vi "Teleop.vi"(10 "Match Info":T1={"Autonomous Elapsed Seconds"=0.0, "TeleOp Elapsed Seconds"=0.0, "Disabled Elapsed Seconds"=0.0, "Visited Autonomous"=FALSE, "Visited TeleOp"=FALSE, "Visited Disabled"=FALSE, "Autonomous Settings"={"Autonomous Style"=enum."Independent", "VI Refnum"=refnum}}, 11 "Call Context":T2) -> ()   [LabVIEW 2017]
doc: "This VI is called for each TeleOp packet received from the DS where the robot is not disabled. It is often used to read from the joysticks and update I/O or to update setpoints for timed control loops. It should complete and return within 20 milliseconds or it may miss DS packets."
uses:
  <vilib>/Rock Robotics/WPI/DriverStation/WPI_DriverStationDerivedRobotMode.ctl
  <vilib>/Rock Robotics/WPI/DriverStation/WPI_DriverStationMatch Info.ctl
  Climb Controls.ctl
  Cube Manipulation Manual Controls.ctl
  Cube Manipulation Controls.ctl
  <vilib>/Rock Robotics/WPI/ThirdParty/Phoenix-LabVIEW/Motor Controller/Controls/CTRE_Phoenix_MotorControl_ControlMode.ctl
  Robot Global Data.vi
  <vilib>/Rock Robotics/WPI/Utilities/WPI_GetSetVariantRefNum.vi
  <vilib>/Rock Robotics/WPI/Solenoid/Deprecated/WPI_SolenoidSetBool.vi
  <vilib>/Rock Robotics/WPI/Solenoid/Deprecated/WPI_SolenoidGetBool.vi
panel:
  out "Ramp Tail":bool
  out "Ramp Drop":bool
  in  "Carrage Contiunous voltage":dbl=-1.0
  in  "Swerve Debug Mode":bool
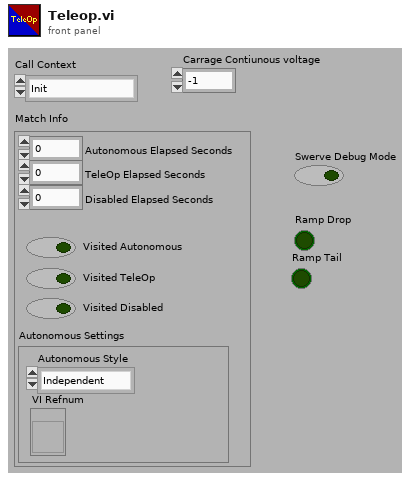
[diagram p1: front panel]
types:
  T1 = typedef "WPI_DriverStationMatch Info.ctl" = cluster{"Autonomous Elapsed Seconds":dbl, "TeleOp Elapsed Seconds":dbl, "Disabled Elapsed Seconds":dbl, "Visited Autonomous":bool, "Visited TeleOp":bool, "Visited Disabled":bool, "Autonomous Settings":cluster{"Autonomous Style":enum16{"Iterative", "Independent"}, "VI Refnum":refnum<vi>}}
  T2 = typedef "WPI_DriverStationDerivedRobotMode.ctl" = enum16{"Init", "Execute", "Stop"}
  T3 = typedef "Cube Manipulation Controls.ctl" = cluster{"Intake Sequence":bool, "Switch Position":bool, "Scale Position Low":bool, "Scale Position Mid":bool, "Scale Position High":bool, "Re-adjust Grip":bool, "Manual Mode":bool, "Manual Toggle Long":bool, "Manual Toggle Short":bool, "Eject Cube":bool, "Manual Lift Control":bool, "Exchange Sequence":bool, "Open Intk Short 4 Intk":bool, "Slow Eject":bool}
  T4 = typedef "Cube Manipulation Manual Controls.ctl" = cluster{"Extend Long Solinoid":bool, "Retract Long Solinoid":bool, "Extend Short Solinoid":bool, "Retract Short Solinoid":bool, "Override Lift Control":bool, "Override Intake Control":bool, "Clear Intake Area":bool}
  T5 = typedef "Climb Controls.ctl" = cluster{"Drop Ramps":bool, "Lift to Climb":bool, "Attach Hooks":bool, "Extend Ramp Tail":bool, "Climb Output":dbl, "Lift to Cube Hold":bool, "Retract Ramp Tail":bool, "Retract Hooks":bool, "Slack Out of Climb":bool, "Slack Out of Climb R":bool}
  T6 = typedef "WPI_JoystickDevRef.ctl" = cluster{"Device":T7}
  T7 = typedef "WPI_JoystickDeviceEnum.ctl" = enum16{"USB 0", "USB 1", "USB 2", "USB 3", "USB 4", "USB 5"}
  T8 = typedef "Cube Manipulation Outputs.ctl" = cluster{"Control Mode":T9, "Carrage Output":dbl, "Intake Output":dbl, "Intake Short":bool, "Intake Long":bool, "Lift Output":dbl, "Lift Output L":dbl, "Lift Output R":dbl}
  T9 = typedef "CTRE_Phoenix_MotorControl_ControlMode.ctl" = u16
  T10 = typedef "Climb Outputs.ctl" = cluster{"Ramp Drop":bool, "Ramp Tail":bool, "Climb Output":dbl, "Lift Output":dbl, "Position Control Mode":bool, "Hook Deploy":bool, "Lift Decend":bool}
  T11 = typedef "WPI_ServoDeviceRef.ctl" = cluster{"DeviceStatus":errorcluster, "PWM Channel":T12, "DeadBand":T13}
  T12 = typedef "FPGA_DIOPWMChannel.ctl" = enum8{"PWM 0", "PWM 1", "PWM 2", "PWM 3", "PWM 4", "PWM 5", "PWM 6", "PWM 7", "PWM 8", "PWM 9", "PWM MXP 0", "PWM MXP 1", "PWM MXP 2", "PWM MXP 3", "PWM MXP 4", "PWM MXP 5", "PWM MXP 6", "PWM MXP 7", "PWM MXP 8", "PWM MXP 9", "Invalid"}
  T13 = typedef "WPI_PWMDeadband.ctl" = cluster{"Name":string, "maxPositivePwm":i32, "minPositivePwm":i32, "centerPwm":i32, "maxNegativePwm":i32, "minNegativePwm":i32, "angularRange":u16}
  T14 = typedef "WPI_SolenoidDevRef.ctl" = cluster{"DevStatus":errorcluster, "Pneumatics Control Module":u8, "Forward Solenoid Channel":T15, "Reverse Solenoid Channel":T15}
  T15 = typedef "WPI_SolenoidChannel.ctl" = enum8{"Solenoid 0", "Solenoid 1", "Solenoid 2", "Solenoid 3", "Solenoid 4", "Solenoid 5", "Solenoid 6", "Solenoid 7", "Invalid"}
  T16 = typedef "WPI_MotorControlDeviceRef.ctl" = cluster{"DeviceStatus":errorcluster, "Type":T17, "PWM":cluster{"PWM Channel":T12, "DeadBand":T13}, "CAN":cluster{"Device Number":u8, "SetOutput VI Ref":variant, "GetOutput VI Ref":variant, "Enable VI Ref":variant, "Disable VI Ref":variant, "Data":variant}, "Invert":bool, "DIO PWM":cluster{"PWM \"Enable\" Channel":T12, "DIOChannel":T18, "PWM Rate":dbl}}
  T17 = typedef "WPI_MotorControlType.ctl" = enum16{"PWM", "CAN", "DIO PWM"}
  T18 = typedef "FPGA_DIOChannel.ctl" = enum8{"DIO 0", "DIO 1", "DIO 2", "DIO 3", "DIO 4", "DIO 5", "DIO 6", "DIO 7", "DIO 8", "DIO 9", "DIO MXP 0", "DIO MXP 1", "DIO MXP 2", "DIO MXP 3", "DIO MXP 4", "DIO MXP 5", "DIO MXP 6", "DIO MXP 7", "DIO MXP 8", "DIO MXP 9", "DIO MXP 10", "DIO MXP 11", "DIO MXP 12", "DIO MXP 13", "DIO MXP 14", "DIO MXP 15", "SPI Port CS1", "SPI Port CS2", "SPI Port CS3", "SPI Port MISO", "SPI Port MOSI", "Invalid"}
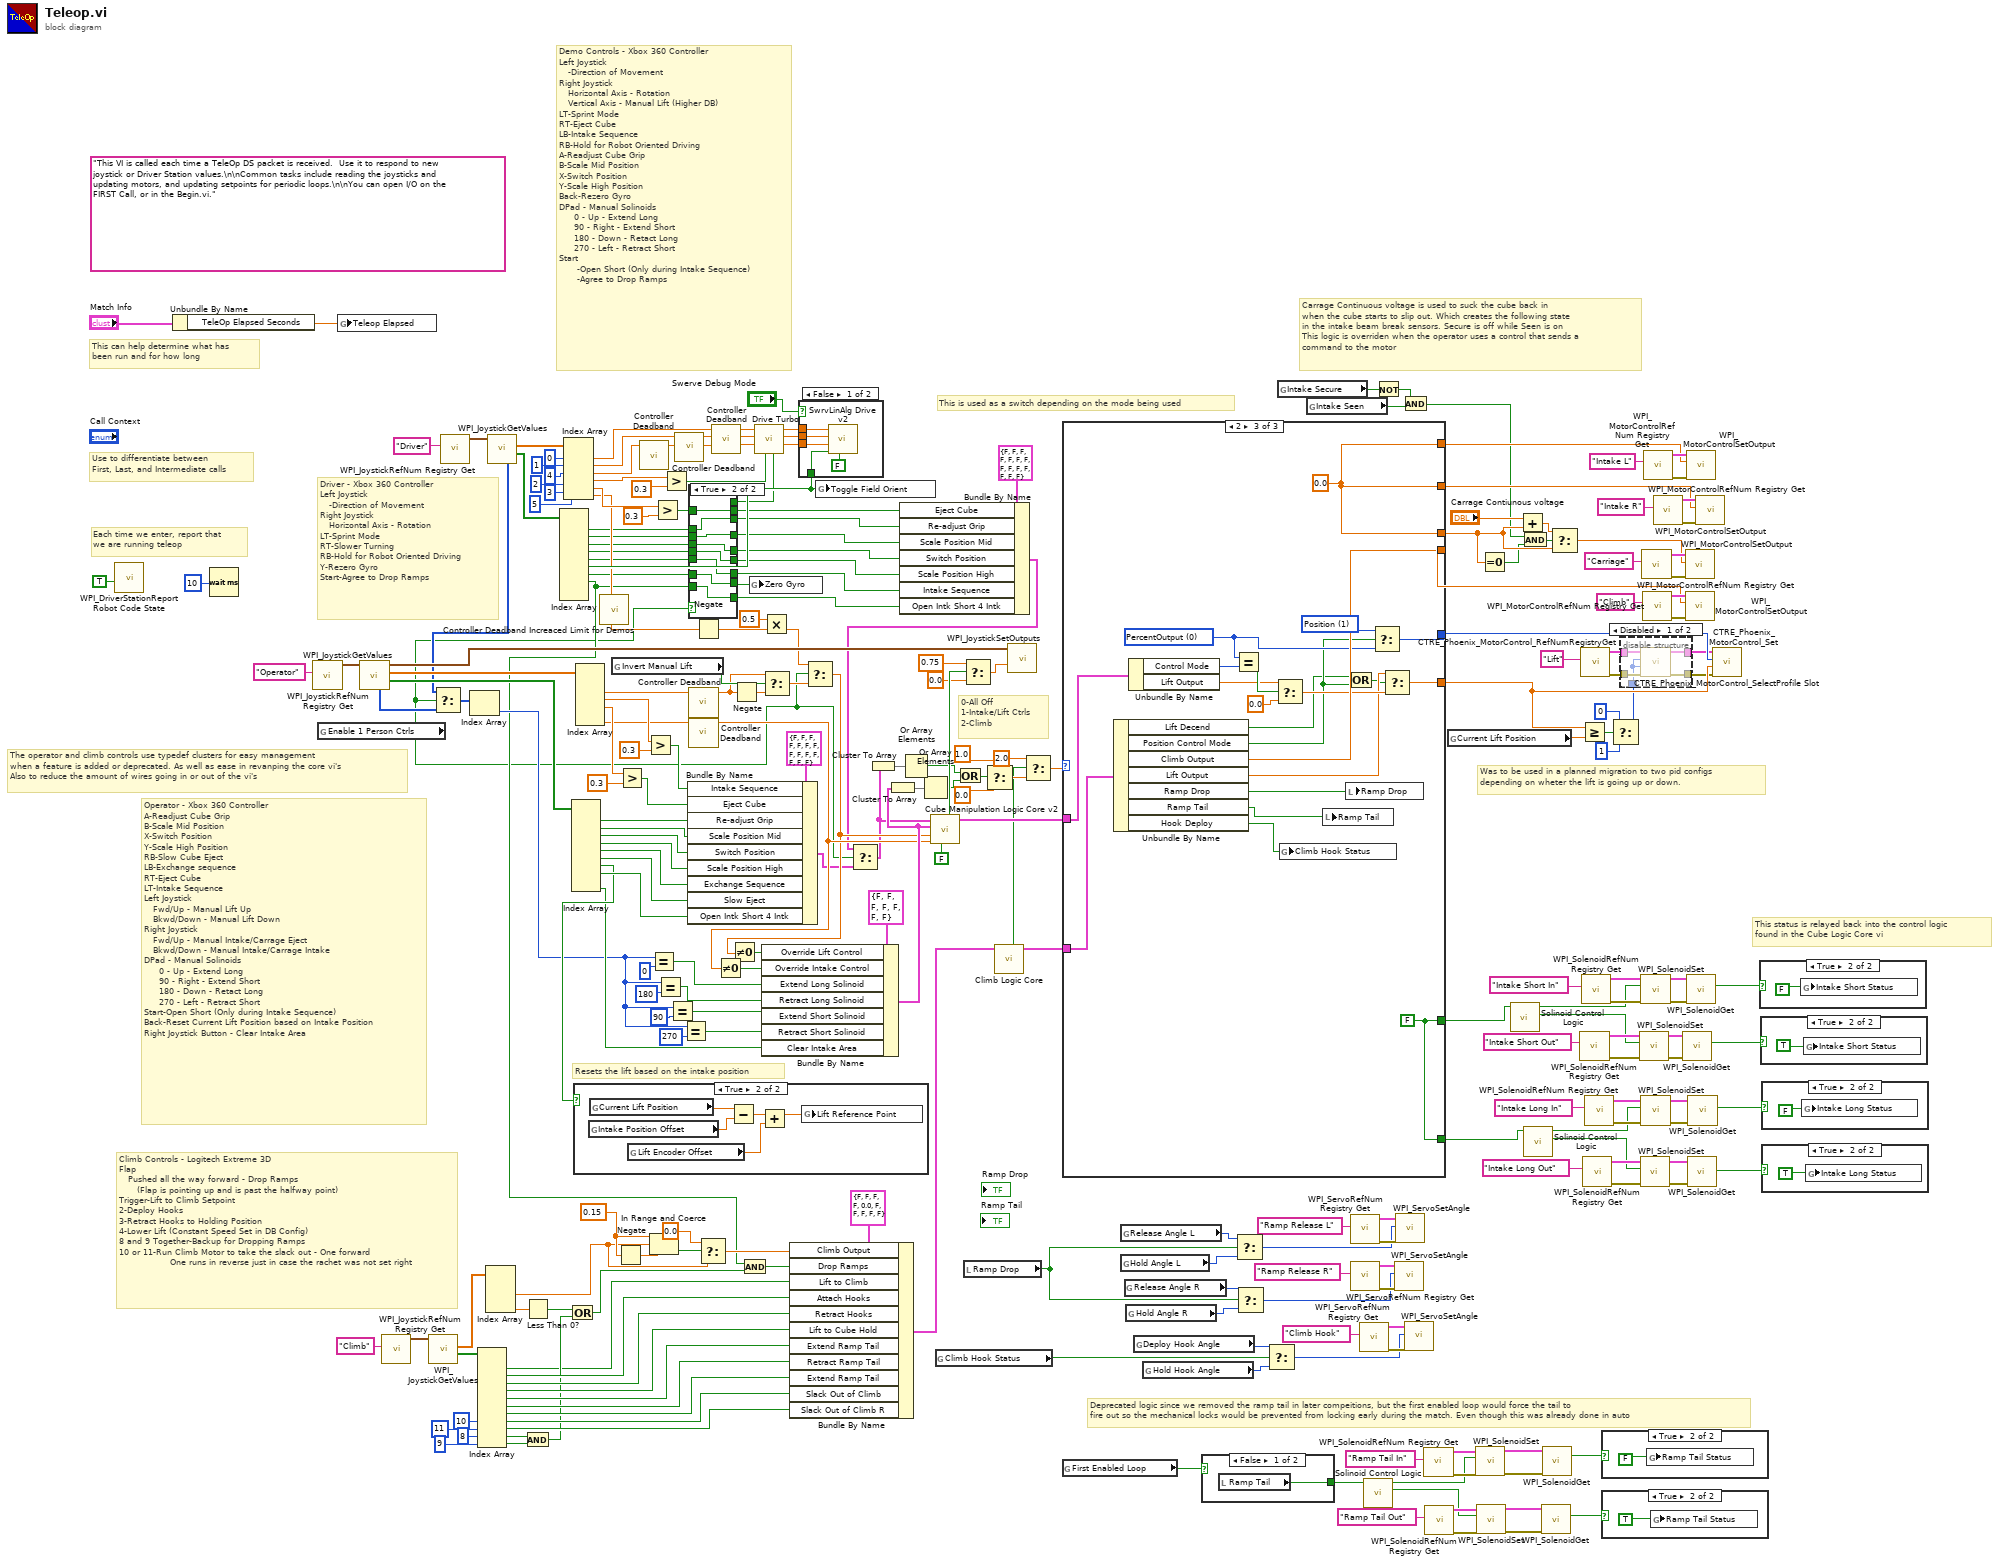
[diagram p0: block diagram]
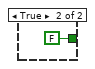
[diagram p4: hidden frame]
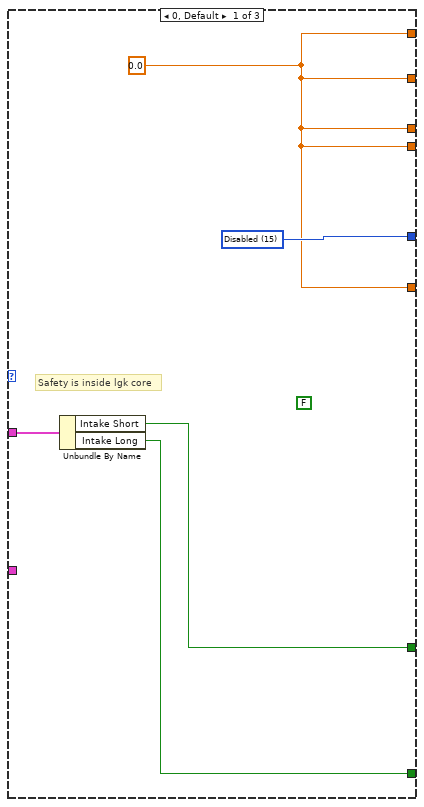
[diagram p12: hidden frame]
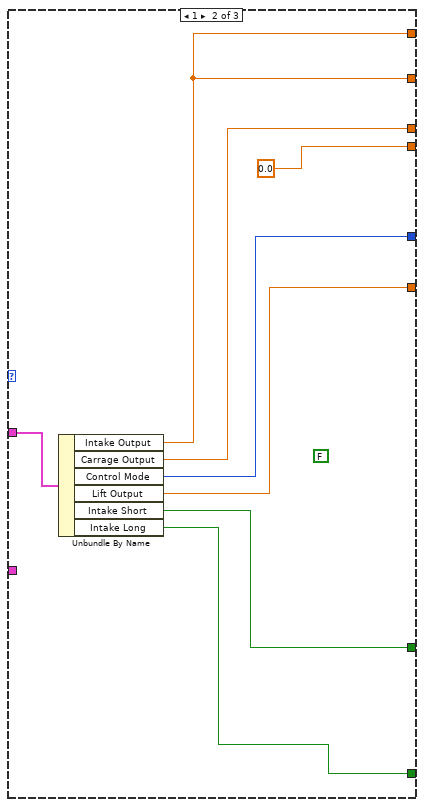
[diagram p13: hidden frame]
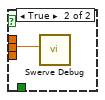
[diagram p14: hidden frame]
diagram:
  w171 = 0.15 ("upper limit")
  (unwired) "This VI is called each time a TeleOp DS packet is received.  Use it to respond to new joystick or Driver Station values.\n\nCommon tasks include reading the joysticks and updating motors, and updating setpoints for periodic loops.\n\nYou can open I/O on the FIRST Call, or in the Begin.vi."
  # "Demo Controls - Xbox 360 Controller\nLeft Joystick \n   -Direction of Movement\nRight Joystick\n   Horizontal Axis - Rotation\n   Vertical Axis - Manual Lift (Higher DB)\nLT-Sprint Mode\nRT-Eject Cube\nLB-Intake Sequence\nRB-Hold for Robot Oriented Driving\nA-Readjust Cube Grip\nB-Scale Mid Position\nX-Switch Position\nY-Scale High Position\nBack-Rezero Gyro\nDPad - Manual Solinoids\n     0 - Up - Extend Long\n     90 - Right - Extend Short\n     180 - Down - Retact Long\n     270 - Left - Retract Short\nStart\n      -Open Short (Only during Intake Sequence)\n      -Agree to Drop Ramps"
  # "Deprecated logic since we removed the ramp tail in later compeitions, but the first enabled loop would force the tail to \nfire out so the mechanical locks would be prevented from locking early during the match. Even though this was already done in auto"
  # "Was to be used in a planned migration to two pid configs\ndepending on wheter the lift is going up or down."
  # "This status is relayed back into the control logic\nfound in the Cube Logic Core vi"
  # "Carrage Continuous voltage is used to suck the cube back in\nwhen the cube starts to slip out. Which creates the following state\nin the intake beam break sensors. Secure is off while Seen is on\nThis logic is overriden when the operator uses a control that sends a \ncommand to the motor"
  # "This is used as a switch depending on the mode being used"
  # "The operator and climb controls use typedef clusters for easy management\nwhen a feature is added or deprecated. As well as ease in revanping the core vi's \nAlso to reduce the amount of wires going in or out of the vi's"
  # "Driver - Xbox 360 Controller\nLeft Joystick \n   -Direction of Movement\nRight Joystick\n   Horizontal Axis - Rotation\nLT-Sprint Mode\nRT-Slower Turning\nRB-Hold for Robot Oriented Driving\nY-Rezero Gyro\nStart-Agree to Drop Ramps"
  # "Climb Controls - Logitech Extreme 3D\nFlap\n   Pushed all the way forward - Drop Ramps\n      (Flap is pointing up and is past the halfway point)\nTrigger-Lift to Climb Setpoint\n2-Deploy Hooks\n3-Retract Hooks to Holding Position\n4-Lower Lift (Constant Speed Set in DB Config)\n8 and 9 Together-Backup for Dropping Ramps\n10 or 11-Run Climb Motor to take the slack out - One forward\n                 One runs in reverse just in case the rachet was not set right"
  # "Resets the lift based on the intake position"
  # "Operator - Xbox 360 Controller\nA-Readjust Cube Grip\nB-Scale Mid Position\nX-Switch Position\nY-Scale High Position\nRB-Slow Cube Eject\nLB-Exchange sequence\nRT-Eject Cube\nLT-Intake Sequence\nLeft Joystick \n   Fwd/Up - Manual Lift Up\n   Bkwd/Down - Manual Lift Down \nRight Joystick \n   Fwd/Up - Manual Intake/Carrage Eject \n   Bkwd/Down - Manual Intake/Carrage Intake\nDPad - Manual Solinoids\n     0 - Up - Extend Long\n     90 - Right - Extend Short\n     180 - Down - Retact Long\n     270 - Left - Retract Short\nStart-Open Short (Only during Intake Sequence)\nBack-Reset Current Lift Position based on Intake Position\nRight Joystick Button - Clear Intake Area"
  # "0-All Off\n1-Intake/Lift Ctrls\n2-Climb"
  # "Each time we enter, report that\nwe are running teleop"
  # "Use to differentiate between\nFirst, Last, and Intermediate calls"
  # "This can help determine what has\nbeen run and for how long"
  n1 = call <vilib>:"WPI_DriverStationReport Robot Code State.vi"("TeleOp"=TRUE ("Autonomous")) -> ()  [unwired: 10 in, 1 out]
  n2 = Unbundle By Name("Match Info") -> ("TeleOp Elapsed Seconds"=w190:dbl)
  n3 = Wait (ms)(milliseconds to wait=u32 10) -> ()  [unwired: 1 out]
  n4 = call <vilib>:"WPI_JoystickRefNum Registry Get.vi"("refnum name"="Operator") -> ("JoystickDevRef"=w249:T6)  [unwired: 1 in, 9 out]
  n5 = global read "Robot Global Data.vi" "Enable 1 Person Ctrls"() -> (w4:bool)
  n6 = global write "Robot Global Data.vi" "Teleop Elapsed"(w190) -> ()
  n7 = call <vilib>:"WPI_JoystickGetValues.vi"("JoystickDevRef"=w249) -> ("Buttons"=w242:bool[], "Axes"=w248:dbl[], "JoystickDevRef"=w194:T6, "POVs"=w34:i16[])  [unwired: 6 in, 1 out]
  n8 = call <vilib>:"WPI_JoystickRefNum Registry Get.vi"("refnum name"="Climb") -> ("JoystickDevRef"=w177:T6)  [unwired: 1 in, 9 out]
  n9 = call <vilib>:"WPI_JoystickGetValues.vi"("JoystickDevRef"=w177) -> ("Buttons"=w175:bool[], "Axes"=w176:dbl[])  [unwired: 6 in, 3 out]
  n10 = call <vilib>:"WPI_JoystickRefNum Registry Get.vi"("refnum name"="Driver") -> ("JoystickDevRef"=w253:T6)  [unwired: 1 in, 9 out]
  n11 = Index Array(array=w175, index #8=10 ("index"), index #9=11 ("index"), index #10=8 ("index"), index #11=9 ("index")) -> (element #1=w40:bool, element #2=w125:bool, element #3=w124:bool, element #4=w123:bool, element #5=w122:bool, element #6=w121:bool, element #7=w120:bool, element #8=w51:bool, element #9=w50:bool, element #10=w37:bool, element #11=w36:bool)  [unwired: 7 in]
  n12 = Index Array(array=w176) -> (element #2=w170:dbl, element #4=w46:dbl)  [unwired: 4 in, 2 out]
  n13 = call <vilib>:"WPI_JoystickGetValues.vi"("JoystickDevRef"=w253) -> ("Buttons"=w244:bool[], "Axes"=w251:dbl[], "POVs"=w32:i16[])  [unwired: 6 in, 2 out]
  n14 = Select(t=w32, s=w4, f=w34) -> (s? t:f=w33:i16[])
  n15 = Index Array(array=w33) -> (element=w35:i16)  [unwired: 1 in]
  n16 = Less Than 0?(x=w46) -> (x < 0?=w45:bool)
  n17 = And(x=w37, y=w36) -> (x .and. y?=w44:bool)
  n18 = Index Array(array=w244) -> (element #1=w18:bool, element #2=w16:bool, element #3=w14:bool, element #4=w20:bool, element #5=w11:bool, element #6=w47:bool, element #7=w9:bool, element #8=w8:bool)  [unwired: 10 in, 2 out]
  n19 = Index Array(array=w251, index #1=0 ("index"), index #2=1 ("index"), index #3=4 ("index"), index #4=2 ("index"), index #5=3 ("index"), index #6=5 ("index")) -> (element #1=w238:dbl, element #2=w237:dbl, element #3=w236:dbl, element #4=w195:dbl, element #5=w95:dbl, element #6=w30:dbl)
  n20 = Or(x=w45, y=w44) -> (x .or. y?=w43:bool)
  n21 = Index Array(array=w242) -> (element #1=w223:bool, element #2=w212:bool, element #3=w211:bool, element #4=w222:bool, element #5=w221:bool, element #6=w220:bool, element #7=w53:bool, element #8=w102:bool, element #10=w52:bool)  [unwired: 10 in, 1 out]
  n22 = case shown="True" w53 {
    frame False {
    }
    frame True {
      n23 = global read "Robot Global Data.vi" "Intake Position Offset"() -> (w259:dbl)
      n24 = global read "Robot Global Data.vi" "Current Lift Position"() -> (w258:dbl)
      n25 = global read "Robot Global Data.vi" "Lift Encoder Offset"() -> (w256:dbl)
      n26 = Subtract(x=w258, y=w259) -> (x-y=w260:dbl)
      n27 = Add(x=w260, y=w256) -> (x+y=w257:dbl)
      n28 = global write "Robot Global Data.vi" "Lift Reference Point"(w257) -> ()
    }
  }
  n29 = Index Array(array=w248) -> (element #2=w217:dbl, element #3=w214:dbl, element #4=w213:dbl, element #6=w167:dbl)  [unwired: 6 in, 2 out]
  n30 = call "Controller Deadband Increaced Limit for Demos.vi"("Input"=w30) -> ("Output"=w29:dbl)  [unwired: 10 in]
  n31 = global read "Robot Global Data.vi" "Invert Manual Lift"() -> (w92:bool)
  n32 = Negate(x=w171) -> (-x=w172:dbl)
  n33 = Greater?(x=w213, y=0.3) -> (0:w169:bool)
  n34 = call "Controller Deadband.vi"("Input"=w236) -> ("Output"=w200:dbl)  [unwired: 10 in]
  n35 = Greater?(x=w214, y=0.3) -> (0:w168:bool)
  n36 = Equal?(x=w35, y=i16 0) -> (x = y?=w158:bool)
  n37 = In Range and Coerce(upper limit=w171, x=w170, lower limit=w172) -> (In Range?=w173:bool)  [unwired: 1 out]
  n38 = Greater?(x=w95, y=0.3) -> (0:w23:bool)
  n39 = Equal?(x=w35, y=i16 180) -> (x = y?=w161:bool)
  n40 = Greater?(x=w195, y=0.3) -> (0:w94:bool)
  n41 = Equal?(x=w35, y=i16 90) -> (x = y?=w160:bool)
  n42 = call "Controller Deadband.vi"("Input"=w237) -> ("Output"=w199:dbl)  [unwired: 10 in]
  n43 = Equal?(x=w35, y=i16 270) -> (x = y?=w159:bool)
  n44 = Bundle By Name(cluster=T3 {"Intake Sequence"=FALSE, "Switch Position"=FALSE, "Scale Position Low"=FALSE, "Scale Position Mid"=FALSE, "Scale Position High"=FALSE, "Re-adjust Grip"=FALSE, "Manual Mode"=FALSE, "Manual Toggle Long"=FALSE, "Manual Toggle Short"=FALSE, "Eject Cube"=FALSE, "Manual Lift Control"=FALSE, "Exchange Sequence"=FALSE, "Open Intk Short 4 Intk"=FALSE, "Slow Eject"=FALSE} ("Cube Button Controls"), "Intake Sequence"=w168, "Eject Cube"=w169, "Re-adjust Grip"=w223, "Scale Position Mid"=w212, "Switch Position"=w211, "Scale Position High"=w222, "Exchange Sequence"=w221, "Slow Eject"=w220, "Open Intk Short 4 Intk"=w102) -> (w5:T3)
  n45 = case shown="True" w4 {
    tunnel: w23 -> [w262 w270]
    tunnel: [w262 _] -> w22
    tunnel: [_ w270] -> w21
    tunnel: w20 -> [w261 w266]
    tunnel: [w261 w264] -> w19
    tunnel: w18 -> [_ w269]
    tunnel: [_ w269] -> w17
    tunnel: w16 -> [_ w268]
    tunnel: [_ w268] -> w15
    tunnel: w14 -> [_ w267]
    tunnel: [_ w267] -> w13
    tunnel: [_ w266] -> w12
    tunnel: w11 -> [_ w265]
    tunnel: [_ w265] -> w10
    tunnel: w9 -> [_ w264]
    tunnel: w8 -> [_ w263]
    tunnel: [_ w263] -> w7
    frame False {
    }
    frame True {
    }
  }
  n46 = call "Controller Deadband.vi"("Input"=w217) -> ("Output"=w54:dbl)  [unwired: 10 in]
  n47 = call "Controller Deadband.vi"("Input"=w167) -> ("Output"=w28:dbl)  [unwired: 10 in]
  n48 = Negate(x=w29) -> (-x=w25:dbl)
  n49 = Select(t=0.0, s=w173, f=w170) -> (s? t:f=w42:dbl)
  n50 = call "Controller Deadband.vi"("Input"=w238) -> ("Output"=w198:dbl)  [unwired: 10 in]
  n51 = Not Equal To 0?(x=w28) -> (x != 0?=w164:bool)
  n52 = Negate(x=w54) -> (-x=w55:dbl)
  n53 = And(x=w8, y=w43) -> (x .and. y?=w41:bool)
  n54 = global write "Robot Global Data.vi" "Zero Gyro"(w19) -> ()
  n55 = call "Drive Turbo.vi"("Slow Rotation"=w22, "Turbo"=w94, "Z"=w200, "Y"=w199, "X"=w198) -> ("Z 2"=w201:dbl, "Y 2"=w202:dbl, "X 2"=w203:dbl)  [unwired: 4 in]
  n56 = Multiply(x=0.5, y=w25) -> (x*y=w2:dbl)
  n57 = Select(t=w54, s=w92, f=w55) -> (s? t:f=w27:dbl)
  n58 = Bundle By Name(cluster=T5 {"Drop Ramps"=FALSE, "Lift to Climb"=FALSE, "Attach Hooks"=FALSE, "Extend Ramp Tail"=FALSE, "Climb Output"=0.0, "Lift to Cube Hold"=FALSE, "Retract Ramp Tail"=FALSE, "Retract Hooks"=FALSE, "Slack Out of Climb"=FALSE, "Slack Out of Climb R"=FALSE} ("Climb Controls"), "Climb Output"=w42, "Drop Ramps"=w41, "Lift to Climb"=w40, "Attach Hooks"=w125, "Retract Hooks"=w124, "Lift to Cube Hold"=w123, "Extend Ramp Tail"=w122, "Retract Ramp Tail"=w121, "Extend Ramp Tail"=w120, "Slack Out of Climb"=w51, "Slack Out of Climb R"=w50) -> (w204:T5)
  n59 = case shown="False" "Swerve Debug Mode" {
    tunnel: w201 -> [w275 _]
    tunnel: w202 -> [w274 w276]
    tunnel: w203 -> [w273 _]
    tunnel: w47 -> [w272 _]
    frame False {
      n60 = call "SwrvLinAlg Drive v2.vi"("Auto Controls"=FALSE, "Robot-Centric"=w272, "Z"=w275, "Y"=w274, "X"=w273) -> ()  [unwired: 7 in]
    }
    frame True {
      n61 = call "Swerve Debug.vi"("Controller"=w276) -> ()  [unwired: 11 in]
    }
  }
  n62 = Select(t=w2, s=w4, f=w27) -> (s? t:f=w26:dbl)
  n63 = Not Equal To 0?(x=w26) -> (x != 0?=w165:bool)
  n64 = Bundle By Name(cluster=T4 {"Extend Long Solinoid"=FALSE, "Retract Long Solinoid"=FALSE, "Extend Short Solinoid"=FALSE, "Retract Short Solinoid"=FALSE, "Override Lift Control"=FALSE, "Override Intake Control"=FALSE, "Clear Intake Area"=FALSE} ("Cube Manipulation Manual Controls"), "Override Lift Control"=w165, "Override Intake Control"=w164, "Extend Long Solinoid"=w158, "Retract Long Solinoid"=w161, "Extend Short Solinoid"=w160, "Retract Short Solinoid"=w159, "Clear Intake Area"=w52) -> (w114:T4)
  n65 = global write "Robot Global Data.vi" "Toggle Field Orient"(w47) -> ()
  n66 = Cluster To Array(cluster=w114) -> (array=w157:bool[])
  n67 = Bundle By Name(cluster=T3 {"Intake Sequence"=FALSE, "Switch Position"=FALSE, "Scale Position Low"=FALSE, "Scale Position Mid"=FALSE, "Scale Position High"=FALSE, "Re-adjust Grip"=FALSE, "Manual Mode"=FALSE, "Manual Toggle Long"=FALSE, "Manual Toggle Short"=FALSE, "Eject Cube"=FALSE, "Manual Lift Control"=FALSE, "Exchange Sequence"=FALSE, "Open Intk Short 4 Intk"=FALSE, "Slow Eject"=FALSE} ("Cube Button Controls"), "Eject Cube"=w21, "Re-adjust Grip"=w17, "Scale Position Mid"=w15, "Switch Position"=w13, "Scale Position High"=w12, "Intake Sequence"=w10, "Open Intk Short 4 Intk"=w7) -> (w3:T3)
  n68 = Select(t=w3, s=w4, f=w5) -> (s? t:f=w6:T3)
  n69 = Cluster To Array(cluster=w6) -> (array=w210:bool[])
  n70 = Or Array Elements(Boolean array=w210) -> (logical OR=w154:bool)
  n71 = Or Array Elements(Boolean array=w157) -> (logical OR=w155:bool)
  n72 = call "Cube Manipulation Logic Core v2.vi"("Auto Control"=FALSE, "Manual Intake Control"=w28, "Manual Lift Control"=w26, "Cube Manipulation Manual Controls"=w114, "Cube Manipulation Button Controls"=w6) -> ("output cluster"=w224:T8, "Sequence Done"=w193:bool)  [unwired: 4 in, 1 out]
  n73 = global read "Robot Global Data.vi" "Climb Hook Status"() -> (w58:bool)
  n74 = Or(x=w154, y=w155) -> (x .or. y?=w156:bool)
  n75 = Select(t=0.75, s=w193, f=0.0) -> (s? t:f=w93:dbl)
  n76 = local read "Ramp Drop"() -> (w56:bool)
  n77 = Select(t=1.0, s=w156, f=0.0) -> (s? t:f=w208:dbl)
  n78 = call "Climb Logic Core.vi"("Climb Controls"=w204) -> ("Climb Outputs"=w119:T10, "Climbing Override"=w206:bool)  [unwired: 9 in]
  n79 = call <vilib>:"WPI_JoystickSetOutputs.vi"("Right Rumble"=w93, "JoystickDevRef"=w194) -> ()  [unwired: 8 in, 2 out]
  n80 = Select(t=2.0, s=w206, f=w208) -> (s? t:f=w209:dbl)
  n81 = global read "Robot Global Data.vi" "First Enabled Loop"() -> (w59:bool)
  n82 = case shown="2" w209 {
    tunnel: [w277 w282 w297] -> w228
    tunnel: [w277 w287 w297] -> w101
    tunnel: [w281 w286 w298] -> w113
    tunnel: [w277 w285 w301] -> w112
    tunnel: [w279 w284 w293] -> w227
    tunnel: [w278 w283 w293] -> w226
    tunnel: [w277 0.0 w309] -> w225
    tunnel: w224 -> [w280 w288 w308]
    tunnel: w119 -> [_ _ w310]
    tunnel: [w277 w282 w297] -> w115
    frame 0, Default {
      (unwired) FALSE ("Ramp Tail")
      w281 = T9 15 items=["PercentOutput"=0, "Position"=1, "Velocity"=2, "Current"=3, "Follower"=5, "MotionProfile"=6, "MotionMagic"=7, "MotionMagicArc"=8, "MotionProfileArc"=10, "Disabled"=15] ("Control Mode")
      w277 = 0.0
      # "Safety is inside lgk core"
      n83 = Unbundle By Name(w280) -> ("Intake Short"=w279:bool, "Intake Long"=w278:bool)
    }
    frame 1 {
      (unwired) FALSE ("Ramp Tail")
      n84 = Unbundle By Name(w288) -> ("Intake Output"=w282:dbl, "Carrage Output"=w287:dbl, "Control Mode"=w286:T9, "Lift Output"=w285:dbl, "Intake Short"=w284:bool, "Intake Long"=w283:bool)
    }
    frame 2 {
      w293 = FALSE ("Intake Short")
      w299 = T9 1 items=["PercentOutput"=0, "Position"=1, "Velocity"=2, "Current"=3, "Follower"=5, "MotionProfile"=6, "MotionMagic"=7, "MotionMagicArc"=8, "MotionProfileArc"=10, "Disabled"=15] ("t")
      w300 = T9 0 items=["PercentOutput"=0, "Position"=1, "Velocity"=2, "Current"=3, "Follower"=5, "MotionProfile"=6, "MotionMagic"=7, "MotionMagicArc"=8, "MotionProfileArc"=10, "Disabled"=15] ("Control Mode")
      w297 = 0.0
      n85 = Unbundle By Name(w310) -> ("Lift Decend"=w290:bool, "Position Control Mode"=w291:bool, "Climb Output"=w309:dbl, "Lift Output"=w302:dbl, "Ramp Drop"=w296:bool, "Ramp Tail"=w295:bool, "Hook Deploy"=w294:bool)
      n86 = Unbundle By Name(w308) -> ("Control Mode"=w307:T9, "Lift Output"=w305:dbl)
      n87 = Equal?(x=w300, y=w307) -> (x = y?=w306:bool)
      n88 = Select(t=w305, s=w306, f=0.0 ("t")) -> (s? t:f=w303:dbl)
      n89 = global write "Robot Global Data.vi" "Climb Hook Status"(w294) -> ()
      n90 = local write "Ramp Tail"(w295) -> ()
      n91 = local write "Ramp Drop"(w296) -> ()
      n92 = Or(x=w290, y=w291) -> (x .or. y?=w292:bool)
      n93 = Select(t=w299, s=w291, f=w300) -> (s? t:f=w298:T9)
      n94 = Select(t=w302, s=w292, f=w303) -> (s? t:f=w301:dbl)
    }
  }
  n95 = global read "Robot Global Data.vi" "Release Angle L"() -> (w79:i32)
  n96 = global read "Robot Global Data.vi" "Hold Angle L"() -> (w78:i32)
  n97 = global read "Robot Global Data.vi" "Release Angle R"() -> (w77:i32)
  n98 = global read "Robot Global Data.vi" "Hold Angle R"() -> (w76:i32)
  n99 = global read "Robot Global Data.vi" "Deploy Hook Angle"() -> (w74:i32)
  n100 = global read "Robot Global Data.vi" "Hold Hook Angle"() -> (w75:i32)
  n101 = case shown="False" w59 {
    tunnel: [w311 FALSE ("Ramp Tail Status")] -> w57
    frame False {
      n102 = local read "Ramp Tail"() -> (w311:bool)
    }
    frame True {
    }
  }
  n103 = Select(t=w79, s=w56, f=w78) -> (s? t:f=w85:i32)
  n104 = Select(t=w77, s=w56, f=w76) -> (s? t:f=w84:i32)
  n105 = Select(t=w74, s=w58, f=w75) -> (s? t:f=w80:i32)
  n106 = global read "Robot Global Data.vi" "Intake Secure"() -> (w180:bool)
  n107 = global read "Robot Global Data.vi" "Intake Seen"() -> (w182:bool)
  n108 = call <vilib>:"WPI_ServoRefNum Registry Get.vi"("refnum name"="Ramp Release L") -> ("error out"=w89:errorcluster, "ServoDeviceRef"=w88:T11)  [unwired: 9 in]
  n109 = call <vilib>:"WPI_ServoRefNum Registry Get.vi"("refnum name"="Ramp Release R") -> ("error out"=w86:errorcluster, "ServoDeviceRef"=w87:T11)  [unwired: 9 in]
  n110 = call <vilib>:"WPI_ServoRefNum Registry Get.vi"("refnum name"="Climb Hook") -> ("error out"=w82:errorcluster, "ServoDeviceRef"=w81:T11)  [unwired: 9 in]
  n111 = call "Solinoid Control Logic.vi"("Input"=w57) -> ("Out"=w62:bool, "In"=w63:bool)  [unwired: 9 in]
  n112 = Not(x=w180) -> (.not. x?=w181:bool)
  n113 = call <vilib>:"WPI_ServoSetAngle.vi"("error in (no error)"=w86, "Angle"=w84, "ServoDeviceRef"=w87) -> ()  [unwired: 7 in, 2 out]
  n114 = call <vilib>:"WPI_ServoSetAngle.vi"("error in (no error)"=w89, "Angle"=w85, "ServoDeviceRef"=w88) -> ()  [unwired: 7 in, 2 out]
  n115 = And(x=w181, y=w182) -> (x .and. y?=w99:bool)
  n116 = call <vilib>:"WPI_ServoSetAngle.vi"("error in (no error)"=w82, "Angle"=w80, "ServoDeviceRef"=w81) -> ()  [unwired: 7 in, 2 out]
  n117 = call <vilib>:"WPI_SolenoidRefNum Registry Get.vi"("refnum name"="Ramp Tail In") -> ("error out"=w73:errorcluster, "SolenoidDevRef"=w72:T14)  [unwired: 9 in]
  n118 = call <vilib>:"WPI_SolenoidRefNum Registry Get.vi"("refnum name"="Ramp Tail Out") -> ("error out"=w70:errorcluster, "SolenoidDevRef"=w69:T14)  [unwired: 9 in]
  n119 = global read "Robot Global Data.vi" "Current Lift Position"() -> (w111:dbl)
  n120 = call-poly <vilib>:"WPI_SolenoidSet.vi"("error in (no error)"=w73, "Value"=w63, "SolenoidDevRef"=w72) -> ("error out"=w67:errorcluster, "SolenoidDevRef"=w66:T14)  [unwired: 7 in]
  n121 = call-poly <vilib>:"WPI_SolenoidSet.vi"("error in (no error)"=w70, "Value"=w62, "SolenoidDevRef"=w69) -> ("error out"=w64:errorcluster, "SolenoidDevRef"=w65:T14)  [unwired: 7 in]
  n122 = Equal To 0?(x=w101) -> (x = 0?=w98:bool)
  n123 = call "Solinoid Control Logic.vi"("Input"=w227) -> ("Out"=w126:bool, "In"=w127:bool)  [unwired: 9 in]
  n124 = Add(x="Carrage Contiunous voltage", y=w101) -> (x+y=w184:dbl)
  n125 = And(x=w99, y=w98) -> (x .and. y?=w100:bool)
  n126 = call "Solinoid Control Logic.vi"("Input"=w226) -> ("Out"=w128:bool, "In"=w129:bool)  [unwired: 9 in]
  n127 = call-poly <vilib>:"WPI_SolenoidGet.vi"("error in (no error)"=w64, "SolenoidDevRef"=w65) -> ("Value"=w60:bool)  [unwired: 7 in, 2 out]
  n128 = call-poly <vilib>:"WPI_SolenoidGet.vi"("error in (no error)"=w67, "SolenoidDevRef"=w66) -> ("Value"=w61:bool)  [unwired: 7 in, 2 out]
  n129 = Select(t=w184, s=w100, f=w101) -> (s? t:f=w185:dbl)
  n130 = Greater Or Equal?(x=w112, y=w111) -> (x >= y?=w106:bool)
  n131 = call <vilib>:"WPI_SolenoidRefNum Registry Get.vi"("refnum name"="Intake Short Out") -> ("error out"=w143:errorcluster, "SolenoidDevRef"=w142:T14)  [unwired: 9 in]
  n132 = call "CTRE_Phoenix_MotorControl_RefNumRegistryGet.vi"("refnum name"="Lift") -> ("error out"=w108:errorcluster, "PhoenixMotorControlDevRef"=w107:T16)  [unwired: 9 in]
  n133 = call <vilib>:"WPI_SolenoidRefNum Registry Get.vi"("refnum name"="Intake Short In") -> ("error out"=w145:errorcluster, "SolenoidDevRef"=w144:T14)  [unwired: 9 in]
  n134 = call <vilib>:"WPI_SolenoidRefNum Registry Get.vi"("refnum name"="Intake Long Out") -> ("error out"=w147:errorcluster, "SolenoidDevRef"=w146:T14)  [unwired: 9 in]
  n135 = call <vilib>:"WPI_SolenoidRefNum Registry Get.vi"("refnum name"="Intake Long In") -> ("error out"=w149:errorcluster, "SolenoidDevRef"=w148:T14)  [unwired: 9 in]
  n136 = case shown="True" w61 {
    frame False {
    }
    frame True {
      n137 = global write "Robot Global Data.vi" "Ramp Tail Status"(FALSE ("Intake Long Status")) -> ()
    }
  }
  n138 = case shown="True" w60 {
    frame False {
    }
    frame True {
      n139 = global write "Robot Global Data.vi" "Ramp Tail Status"(TRUE ("Intake Long Status")) -> ()
    }
  }
  n140 = Select(t=0 ("slotIdx"), s=w106, f=1) -> (s? t:f=w103:i32)
  n141 = disable-structure shown="Disabled" {
    disable-tunnel: [w319 w321] -> w110
    disable-tunnel: [w318 w320] -> w109
    disable-tunnel: w108 -> [w317 w320]
    disable-tunnel: w107 -> [w316 w321]
    disable-tunnel: w103 -> [w315 _]
    frame Disabled {
      n142 = call <vilib>:"CTRE_Phoenix_MotorControl_SelectProfile Slot.vi"("error in (no error)"=w317, "pidLoopIdx"=w315, "slotIdx"=w315, "PhoenixMotorControlDevRef"=w316) -> ("error out"=w318:errorcluster, "PhoenixMotorControlDevRef"=w319:T16)  [unwired: 6 in]
    }
    frame Enabled {
    }
  }
  n143 = call-poly <vilib>:"WPI_SolenoidSet.vi"("error in (no error)"=w143, "Value"=w126, "SolenoidDevRef"=w142) -> ("error out"=w135:errorcluster, "SolenoidDevRef"=w134:T14)  [unwired: 7 in]
  n144 = call-poly <vilib>:"WPI_SolenoidSet.vi"("error in (no error)"=w147, "Value"=w128, "SolenoidDevRef"=w146) -> ("error out"=w139:errorcluster, "SolenoidDevRef"=w138:T14)  [unwired: 7 in]
  n145 = call-poly <vilib>:"WPI_SolenoidSet.vi"("error in (no error)"=w145, "Value"=w127, "SolenoidDevRef"=w144) -> ("error out"=w137:errorcluster, "SolenoidDevRef"=w136:T14)  [unwired: 7 in]
  n146 = call-poly <vilib>:"WPI_SolenoidSet.vi"("error in (no error)"=w149, "Value"=w129, "SolenoidDevRef"=w148) -> ("error out"=w141:errorcluster, "SolenoidDevRef"=w140:T14)  [unwired: 7 in]
  n147 = call <vilib>:"WPI_MotorControlRefNum Registry Get.vi"("refnum name"="Carriage") -> ("error out"=w230:errorcluster, "MotorControlDevRef"=w189:T16)  [unwired: 9 in]
  n148 = call <vilib>:"WPI_MotorControlRefNum Registry Get.vi"("refnum name"="Climb") -> ("error out"=w241:errorcluster, "MotorControlDevRef"=w240:T16)  [unwired: 9 in]
  n149 = call <vilib>:"WPI_MotorControlRefNum Registry Get.vi"("refnum name"="Intake L") -> ("error out"=w234:errorcluster, "MotorControlDevRef"=w233:T16)  [unwired: 9 in]
  n150 = call <vilib>:"WPI_MotorControlRefNum Registry Get.vi"("refnum name"="Intake R") -> ("error out"=w118:errorcluster, "MotorControlDevRef"=w117:T16)  [unwired: 9 in]
  n151 = call-poly <vilib>:"WPI_SolenoidGet.vi"("error in (no error)"=w135, "SolenoidDevRef"=w134) -> ("Value"=w132:bool)  [unwired: 7 in, 2 out]
  n152 = call <vilib>:"WPI_MotorControlSetOutput.vi"("error in (no error)"=w230, "Output"=w185, "MotorControlDevRef"=w189) -> ()  [unwired: 6 in, 3 out]
  n153 = call <vilib>:"WPI_MotorControlSetOutput.vi"("error in (no error)"=w241, "Output"=w225, "MotorControlDevRef"=w240) -> ()  [unwired: 6 in, 3 out]
  n154 = call <vilib>:"WPI_MotorControlSetOutput.vi"("error in (no error)"=w234, "Output"=w228, "MotorControlDevRef"=w233) -> ()  [unwired: 6 in, 3 out]
  n155 = call-poly <vilib>:"WPI_SolenoidGet.vi"("error in (no error)"=w137, "SolenoidDevRef"=w136) -> ("Value"=w131:bool)  [unwired: 7 in, 2 out]
  n156 = call-poly <vilib>:"WPI_SolenoidGet.vi"("error in (no error)"=w139, "SolenoidDevRef"=w138) -> ("Value"=w130:bool)  [unwired: 7 in, 2 out]
  n157 = call-poly <vilib>:"WPI_SolenoidGet.vi"("error in (no error)"=w141, "SolenoidDevRef"=w140) -> ("Value"=w133:bool)  [unwired: 7 in, 2 out]
  n158 = call <vilib>:"WPI_MotorControlSetOutput.vi"("error in (no error)"=w118, "Output"=w115, "MotorControlDevRef"=w117) -> ()  [unwired: 6 in, 3 out]
  n159 = call <vilib>:"CTRE_Phoenix_MotorControl_Set.vi"("error in (no error)"=w109, "Output"=w112, "Control Mode"=w113, "PhoenixMotorControlDevRef"=w110) -> ()  [unwired: 6 in, 2 out]
  n160 = case shown="True" w131 {
    frame False {
    }
    frame True {
      n161 = global write "Robot Global Data.vi" "Intake Short Status"(FALSE ("Intake Short Status")) -> ()
    }
  }
  n162 = case shown="True" w132 {
    frame False {
    }
    frame True {
      n163 = global write "Robot Global Data.vi" "Intake Short Status"(TRUE ("Intake Short Status")) -> ()
    }
  }
  n164 = case shown="True" w133 {
    frame False {
    }
    frame True {
      n165 = global write "Robot Global Data.vi" "Intake Long Status"(FALSE ("Intake Long Status")) -> ()
    }
  }
  n166 = case shown="True" w130 {
    frame False {
    }
    frame True {
      n167 = global write "Robot Global Data.vi" "Intake Long Status"(TRUE ("Intake Long Status")) -> ()
    }
  }
